vi "RTM - Remove Unbound Channels.vi"(8 "error in (no error)":errorcluster, 11 "Node Ptr":T1 format="%.0x") -> (0 "error out":errorcluster)   [LabVIEW 2019, in "UDP-Custom-Device System Explorer.lvlib"]
uses:
  UDP-Custom-Device System Explorer.lvlib
  <vilib>/NI VeriStand/Custom Device API/Custom Device Item Ref.ctl
  <vilib>/NI VeriStand/Custom Device Tools/Custom Device Utility Library/Custom Device Utility Library.lvlib
  <vilib>/NI VeriStand/Custom Device API/Custom Device API.lvlib
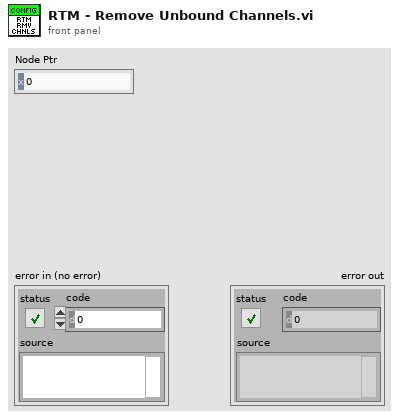
[diagram p1: front panel]
types:
  T1 = typedef "Custom Device API.lvlib/Custom Device Item Ref.ctl" = u64
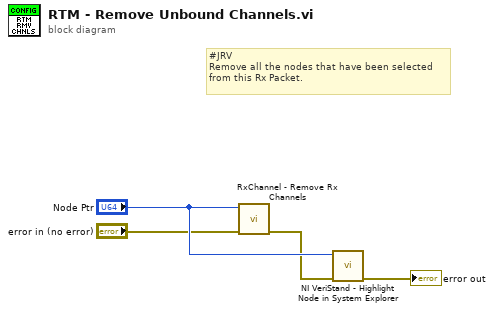
[diagram p0: block diagram]
diagram:
  # "#JRV\nRemove all the nodes that have been selected\nfrom this Rx Packet."
  n1 = call "RxChannel - Remove Rx Channels.vi"("error in (no error)"="error in (no error)", "Node Ptr"="Node Ptr") -> ("error out"=w2:errorcluster)  [unwired: 9 in]
  n2 = call <vilib>:"NI VeriStand - Highlight Node in System Explorer.vi"("error in (no error)"=w2, "Item Ref in"="Node Ptr") -> ("error out"=→"error out":errorcluster)  [unwired: 8 in, 1 out]
